vi "SQLite Insert Template.vi"(8 "error in":errorcluster, 10 "Data":cluster{}, 11 "SQLite Connection in":refnum<class "Connection.lvclass">) -> (0 "error out":errorcluster, 2 "Last INSERT RowID":i64, 3 "SQLite Connection out":refnum<class "Connection.lvclass">)   [LabVIEW 2021]
uses:
  <vilib>/drjdpowell/SQLite Library/SQL Connection/Connection.lvclass
  <vilib>/drjdpowell/SQLite Library/SQL Statement/SQL Statement.lvclass
  <vilib>/drjdpowell/SQLite Library/Transaction Helpers/Transaction.lvlib
  edt.lib/sqlite.lib/EDT SQLite+.lvlib
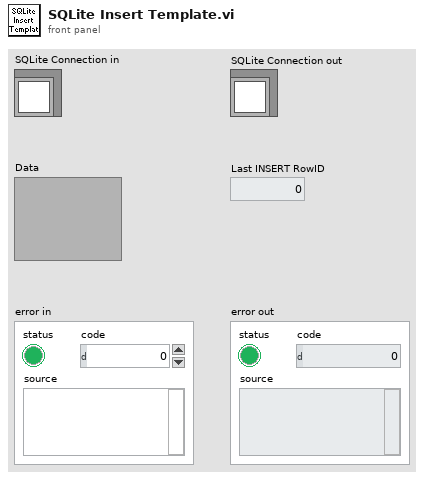
[diagram p1: front panel]
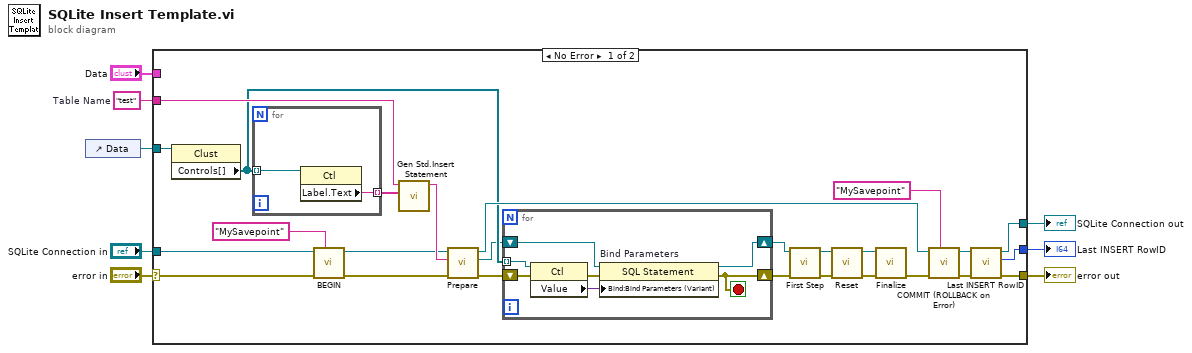
[diagram p0: block diagram]
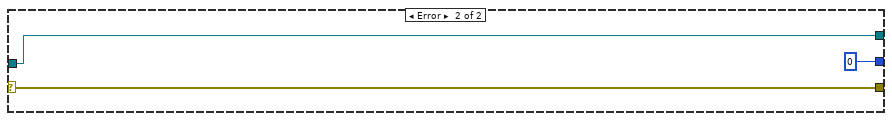
[diagram p2: hidden frame]
diagram:
  w4 = "test"  # Table Name
  n1 = control-ref of="Data"() -> (w2:refnum<vi>)
  n2 = case shown="No Error" "error in" {
    selector: "error in" -> [w27 w46]
    tunnel: [w23 w46] -> w7
    tunnel: "SQLite Connection in" -> [w26 w45]
    tunnel: [w22 w45] -> w5
    tunnel: w4 -> [w20 _]
    tunnel: "Data" -> [_ _]
    tunnel: w2 -> [w17 _]
    tunnel: [w21 i64 0 ("Last INSERT RowID")] -> w1
    frame No Error {
      n3 = property class="Clust"(reference=w17) -> ("Controls[]"=w13:refnum<vi>[])  [unwired: 1 in, 2 out]
      n4 = for {
        tunnel: w13 -> [w43] mode=indexing
        tunnel: [w42] -> w14 mode=indexing
        n5 = property class="Ctl"(reference=w43) -> ("Label.Text"=w42:string)  [unwired: 1 in, 2 out]
      }
      n6 = call <vilib>:"BEGIN.vi"("Savepoint name"="MySavepoint", "error in (no error)"=w27, "SQLite Connection in"=w26) -> ("error out"=w30:errorcluster, "SQLite Connection"=w31:refnum<class "Connection.lvclass">)  [unwired: 7 in]
      n7 = call "Gen Std.Insert Statement.vi"("Field Name"=w14, "Table Name"=w20) -> ("Insert Statement"=w34:string)  [unwired: 9 in]
      n8 = call <vilib>:"Prepare.vi"("error in (no error)"=w30, "SQL"=w34, "SQLite Connection in"=w31) -> ("error out"=w11:errorcluster, "SQL Statement"=w12:refnum<class "SQL Statement.lvclass">, "SQLite Connection"=w29:refnum<class "Connection.lvclass">)  [unwired: 4 in, 2 out]
      n9 = for {
        tunnel: w13 -> [w39] mode=indexing
        shift-right: [w40] -> w9
        shift-left: w12 -> [w38]
        shift-right: [w36] -> w10
        shift-left: w11 -> [w37]
        stop <- w36 stop-if-true
        n10 = property class="Ctl"(reference=w39, error in=w37) -> (error out=w41:errorcluster, "Value"=w35:variant)  [unwired: 1 out]
        n11 = property on="Bind Parameters" class="SQL Statement"(reference=w38, error in=w41, "Bind:Bind Parameters (Variant)"=w35) -> (reference out=w40:refnum<class "SQL Statement.lvclass">, error out=w36:errorcluster)
      }
      n12 = call <vilib>:"First Step.vi"("error in (no error)"=w10, "SQL Statement in"=w9) -> ("error out"=w16:errorcluster, "SQL Statement"=w15:refnum<class "SQL Statement.lvclass">)  [unwired: 7 in, 1 out]
      n13 = call <vilib>:"Reset.vi"("error in (no error)"=w16, "SQL Statement in"=w15) -> ("error out"=w32:errorcluster, "SQL Statement"=w33:refnum<class "SQL Statement.lvclass">)  [unwired: 8 in]
      n14 = call <vilib>:"Finalize.vi"("error in (no error)"=w32, "SQL Statement in"=w33) -> ("error out"=w28:errorcluster)  [unwired: 9 in]
      n15 = call <vilib>:"COMMIT (ROLLBACK on Error).vi"("Savepoint name"="MySavepoint", "error in (no error)"=w28, "SQLite Connection in"=w29) -> ("error out"=w24:errorcluster, "SQLite Connection"=w25:refnum<class "Connection.lvclass">)  [unwired: 7 in]
      n16 = call <vilib>:"Last INSERT RowID.vi"("error in (no error)"=w24, "SQLite Connection in"=w25) -> ("error out"=w23:errorcluster, "Last INSERT RowID"=w21:i64, "SQLite Connection"=w22:refnum<class "Connection.lvclass">)  [unwired: 7 in]
    }
    frame Error {
    }
  }
  "error out" <- w7
  "SQLite Connection out" <- w5
  "Last INSERT RowID" <- w1
